vi "Get Target State.vi"(11 "Transition Command in":refnum<class "Transition Command.lvclass">) -> (2 "Target State":string)   [LabVIEW 2020, in "VolatusSeq.lvlib" / "Transition Command.lvclass"]
uses:
  Transition Command.lvclass
  Transition Command.lvclass/Transition Command.ctl
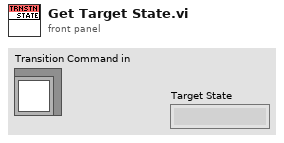
[diagram p1: front panel]
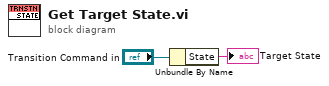
[diagram p0: block diagram]
diagram:
  n1 = Unbundle By Name("Transition Command in") -> ("State"=→"Target State":string)
